vi "ActorEventMessage.vi"(8 "error in (no error)":errorcluster, 9 "Value":string, 10 "Message":string, 11 "UnitTestEngine in":refnum<class "UnitTestEngine.lvclass">) -> (0 "error out":errorcluster, 3 "UnitTestEngine out":refnum<class "UnitTestEngine.lvclass">)   [LabVIEW 2019, in "UnitTestEngine.lvlib" / "UnitTestEngine.lvclass"]
uses:
  UnitTestEngine.lvclass
  UnitTestEngine.lvclass/UnitTestEngine.ctl
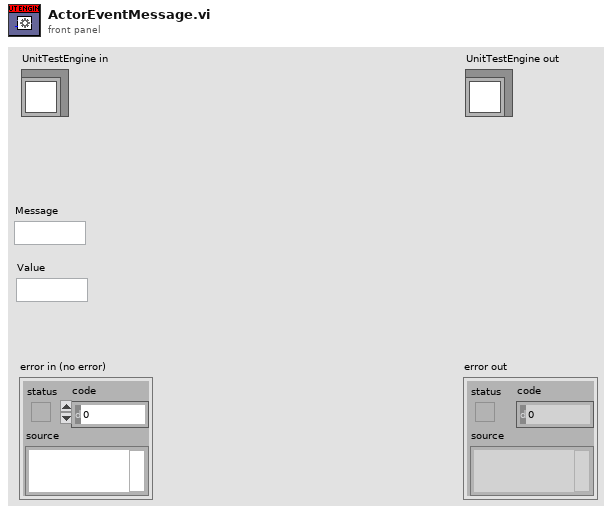
[diagram p1: front panel]
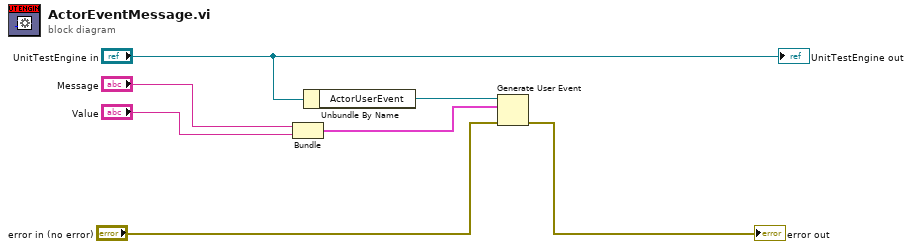
[diagram p0: block diagram]
diagram:
  n1 = Bundle("Message"="Message", "Value"="Value") -> (w6:cluster{"Message":string, "Value":string})  [unwired: 1 in]
  n2 = Unbundle By Name("UnitTestEngine in") -> ("ActorUserEvent"=w7:refnum<user-event>)
  n3 = Generate User Event(user event=w7, event data cluster=w6, error in="error in (no error)") -> (error out=→"error out":errorcluster)  [unwired: 1 in, 1 out]
  "UnitTestEngine out" <- "UnitTestEngine in"
